vi "UnscentedKalmanFilter_GetP.vi"(11 "in UnscentedKalmanFiilter":T2) -> (3 "P":T1)   [LabVIEW 2019, in "Trajectory_Library.lvlib"]
doc: "Returns the error covariance matrix P.\n\nInputs:\n - inUnscentedKalmanFilter -- filter data cluster\n\nOutputs: \n - P -- the error covariance matrix P."
uses:
  Trajectory_Library.lvlib
  UNSCENTED_KALMAN_FILTER.ctl
  <vilib>/Analysis/Matrix/Datatypes/RealMatrix.ctl
  MERWE_SCALED_SIGMA_PTS.ctl
  BiFun_Matrix_FUNC_TYPE.ctl
  <vilib>/Analysis/Matrix/NI_Matrix.lvlib
panel:
  # "State Estimate <Statess,1>"
  # "<States, States>"
  # "<States, ?>"
  # "<Statess,  States>"
  # "<Outputs, Outputs>"
  # "<?, 1>"
  # "<?, 1>"
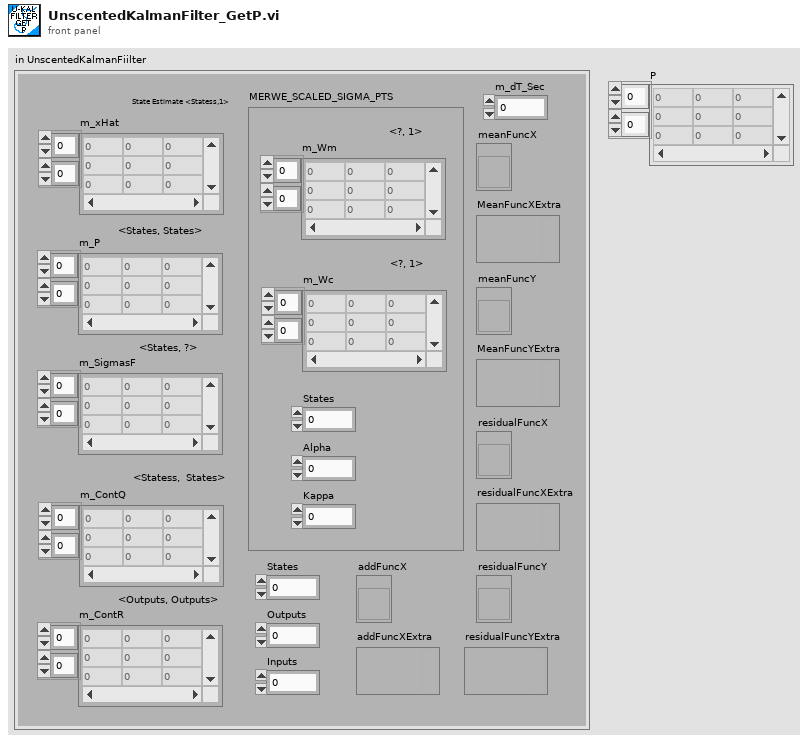
[diagram p1: front panel]
types:
  T1 = typedef "NI_Matrix.lvlib/RealMatrix.ctl" = dbl[][]
  T2 = typedef "Trajectory_Library.lvlib/UNSCENTED_KALMAN_FILTER.ctl" = cluster{"m_P":T1, "m_xHat":T1, "States":i32, "Outputs":i32, "m_ContR":T1, "m_ContQ":T1, "m_SigmasF":T1, "m_dT_Sec":dbl, "MERWE_SCALED_SIGMA_PTS":T3, "meanFuncX":T4, "meanFuncY":T4, "residualFuncX":T4, "residualFuncY":T4, "addFuncX":T4, "addFuncXExtra":variant, "residualFuncYExtra":variant, "residualFuncXExtra":variant, "MeanFuncYExtra":variant, "MeanFuncXExtra":variant, "Inputs":i32}
  T3 = typedef "Trajectory_Library.lvlib/MERWE_SCALED_SIGMA_PTS.ctl" = cluster{"m_Wm":T1, "States":i32, "Alpha":dbl, "m_Wc":T1, "Kappa":i32}
  T4 = typedef "Trajectory_Library.lvlib/BiFun_Matrix_FUNC_TYPE.ctl" = refnum<vi>
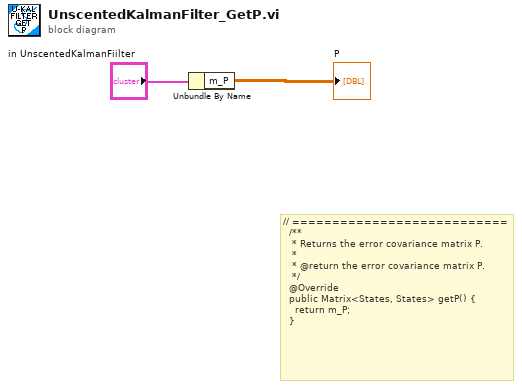
[diagram p0: block diagram]
diagram:
  # "// ===========================\n  /**\n   * Returns the error covariance matrix P.\n   *\n   * @return the error covariance matrix P.\n   */\n  @Override\n  public Matrix<States, States> getP() {\n    return m_P;\n  }"
  n1 = Unbundle By Name("in UnscentedKalmanFiilter") -> ("m_P"=→"P":T1)
